vi "Get Individual Decay Parameters.vi"(8 "Error In":errorcluster, 9 "Global Fit Parameter Info":T1, 10 "# Decays":i32, 11 "Global Fit Parameters Array":dbl[](array[numeric])) -> (0 "Error Out":errorcluster, 1 "Plot Specific Parameters Array":dbl[][](array[numeric]), 2 "Global Parameters":dbl[](array[numeric]), 3 "All Parameters Array":dbl[][](array[numeric]))   [LabVIEW 2021, in "AlliGator Global Decay Fit.lvlib"]
uses:
  Global Fit Parameters Information.ctl
  df948659-0c3b-4728-b540-eef5ddc65b1b.vi
  9c81236d-5440-47e3-bf70-0b74199a9f1c.vi
  2585c82f-6210-440b-b659-fce4af5f9abb.vi
  AlliGator/AlliGator Global Decay Fit.lvlib
  Fits.lvlib
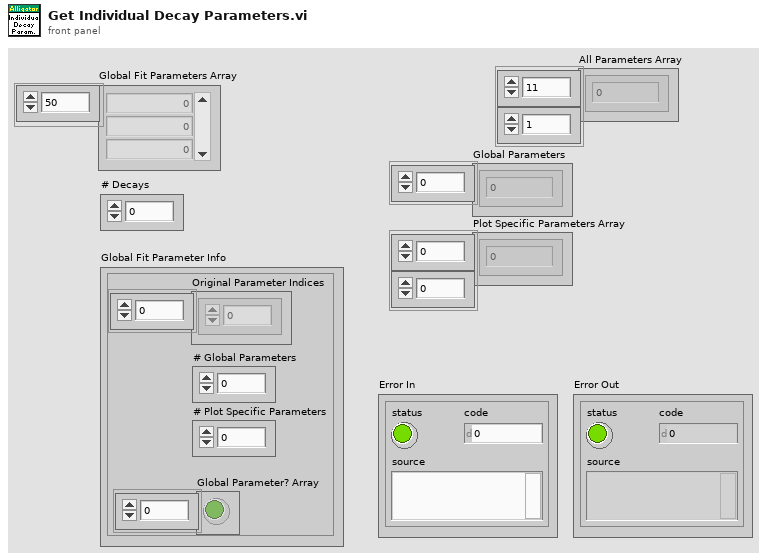
[diagram p1: front panel]
types:
  T1 = typedef "Fits.lvlib/Global Fit Parameters Information.ctl" = cluster{"Original Parameter Indices":i32[], "# Global Parameters":i32, "# Plot Specific Parameters":i32, "Global Parameter? Array":bool[]}
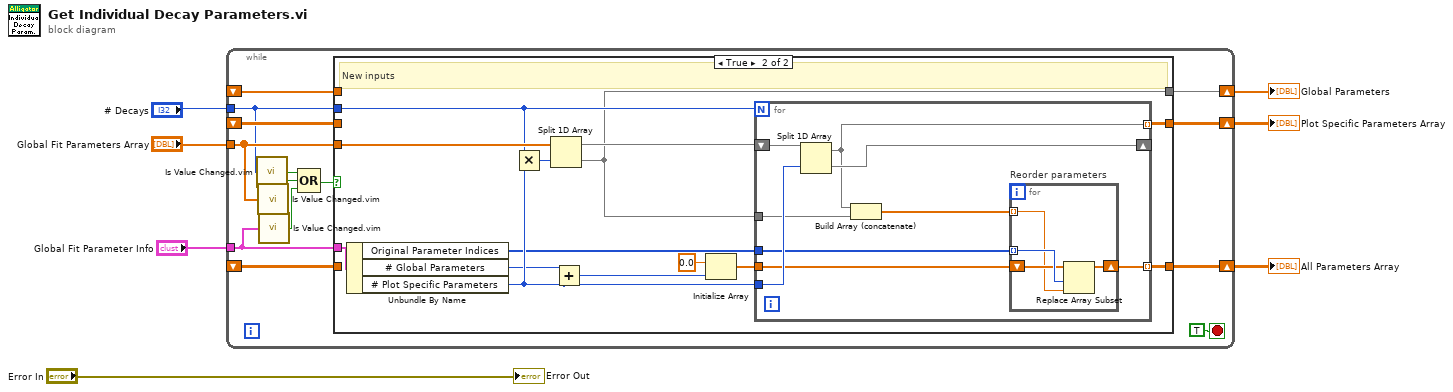
[diagram p0: block diagram]
diagram:
  n1 = while {
    tunnel: "Global Fit Parameter Info" -> [w13]
    tunnel: "# Decays" -> [w12]
    tunnel: "Global Fit Parameters Array" -> [w14]
    shift-right: [w21] -> w4
    shift-left: _ -> [w17]
    shift-right: [w19] -> w1
    shift-left: _ -> [w16]
    shift-right: [w20] -> w3
    shift-left: _ -> [w15]
    stop <- TRUE stop-if-true
    n2 = call "Is Value Changed.vim"("value"=w12) -> ("changed or first call?"=w11:bool)
    n3 = call "Is Value Changed.vim"("value"=w14) -> ("changed or first call?"=w10:bool)
    n4 = call "Is Value Changed.vim"("value"=w13) -> ("changed or first call?"=w9:bool)
    n5 = Compound Arithmetic op=OR(w11, w10, w9) -> (w8:bool)
    n6 = case shown="True" w8 {
      tunnel: w13 -> [_ w38]
      tunnel: w14 -> [_ w34]
      tunnel: w12 -> [_ w32]
      tunnel: [w24 w28] -> w21
      tunnel: [w22 w26] -> w20
      tunnel: [w23 w25] -> w19
      tunnel: w17 -> [w24 _]
      tunnel: w16 -> [w23 _]
      tunnel: w15 -> [w22 _]
      frame False {
        # "No change: no need to recompute"
      }
      frame True {
        # "New inputs"
        n7 = Unbundle By Name(w38) -> ("Original Parameter Indices"=w27:i32[], "# Global Parameters"=w31:i32, "# Plot Specific Parameters"=w33:i32)
        n8 = Multiply(x=w32, y=w33) -> (x*y=w29:i32)
        n9 = Split 1D Array(array=w34, index=w29) -> (first subarray=w30:dbl[], second subarray=w28:dbl[])
        n10 = Add(x=w31, y=w33) -> (x+y=w37:i32)
        n11 = Initialize Array(0.0 ("element"), w37) -> (w35:dbl[])
        n12 = for {
          N: w32 -> [_]
          tunnel: w35 -> [w42]
          shift-right: [w45] -> _
          shift-left: w30 -> [w47]
          tunnel: w33 -> [w46]
          tunnel: w28 -> [w44]
          tunnel: w27 -> [w41]
          tunnel: [w40] -> w26 mode=indexing
          tunnel: [w39] -> w25 mode=indexing
          n13 = Split 1D Array(array=w47, index=w46) -> (first subarray=w39:dbl[], second subarray=w45:dbl[])
          n14 = Build Array (concatenate)(w39, w44) -> (w43:dbl[])
          n15 = for "Reorder parameters" {
            tunnel: w43 -> [w48] mode=indexing
            shift-right: [w49] -> w40
            shift-left: w42 -> [w50]
            tunnel: w41 -> [w51] mode=indexing
            n16 = Replace Array Subset(array=w50, new element=w48, index=w51) -> (w49:dbl[])
          }
        }
      }
    }
  }
  "All Parameters Array" <- w3
  "Global Parameters" <- w4
  "Plot Specific Parameters Array" <- w1
  "Error Out" <- "Error In"
